vi "Configure Trigger.vi"(5 "Trigger Source (0: Internal)":u16(ring) items=["Internal", "External", "Manual", "BUS"], 7 "Channel (1)":i32=1, 8 "error in (no error)":errorcluster, 9 "Point Trigger (F: Disable)":bool, 10 "Continuous Sweep (T: Enable)":bool=TRUE, 11 "VISA resource name":refnum<visa-resource-name>) -> (0 "error out":errorcluster, 3 "VISA resource name out":refnum<visa-resource-name>)   [LabVIEW 2018, in "Agilent ENA Series.lvlib"]
doc: "Configures trigger."
uses:
  Agilent ENA Series.lvlib
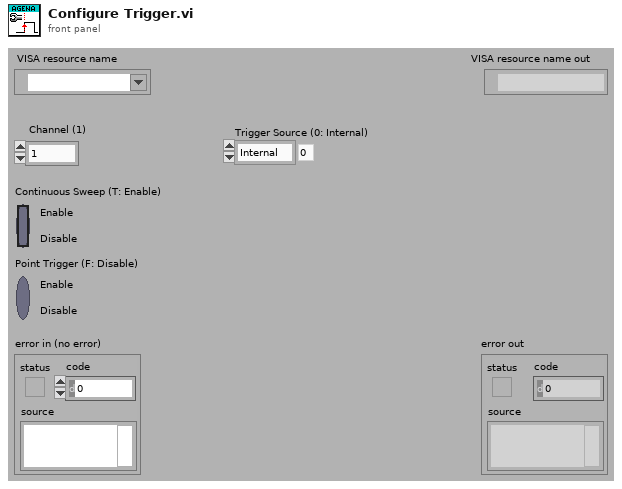
[diagram p1: front panel]
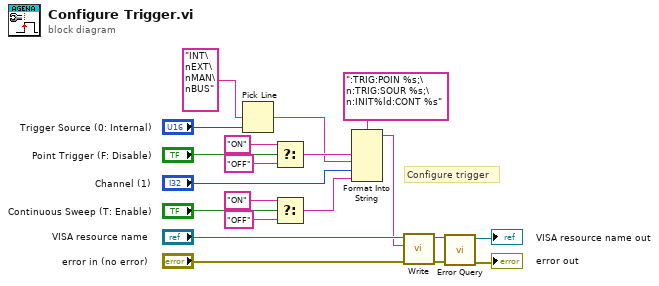
[diagram p0: block diagram]
diagram:
  # "Configure trigger"
  n1 = Pick Line(multi-line string="INT\nEXT\nMAN\nBUS", line index="Trigger Source (0: Internal)") -> (output string=w7:string)  [unwired: 1 in]
  n2 = Select(t="ON", s="Point Trigger (F: Disable)", f="OFF") -> (s? t:f=w9:string)
  n3 = Select(t="ON", s="Continuous Sweep (T: Enable)", f="OFF") -> (s? t:f=w5:string)
  n4 = Format Into String(format string=":TRIG:POIN %s;\n:TRIG:SOUR %s;\n:INIT%ld:CONT %s", w9, w7, "Channel (1)", w5) -> (resulting string=w15:string)  [unwired: 2 in, 1 out]
  n5 = call "Write.vi"("error in (no error)"="error in (no error)", "String ()"=w15, "VISA resource name"="VISA resource name") -> ("error out"=w3:errorcluster, "VISA resource name out"=w4:refnum<visa-resource-name>)  [unwired: 6 in, 1 out]
  n6 = call "Error Query.vi"("error in (no error)"=w3, "VISA resource name"=w4) -> ("error out"=→"error out":errorcluster, "VISA resource name out"=→"VISA resource name out":refnum<visa-resource-name>)  [unwired: 6 in, 2 out]
